vi "multiplier color to multiplier value converter.vi"(2 "mult color":T1) -> (6 "multiplier":dbl)   [LabVIEW 2018]
uses:
  Multiplier--control.ctl
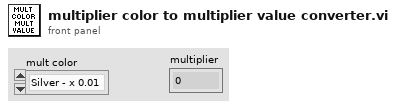
[diagram p1: front panel]
types:
  T1 = typedef "Multiplier--control.ctl" = enum16{"Silver - x 0.01", "Gold - x 0.1 ", "Black - x 1", "Brown - x 10", "Red - x 100", "Orange - x 1k", "Yellow - x 10k", "Green - 100k", "Blue - x 1M", "Violet - x10 M", "Grey - x 100M", "White - x 1G"}
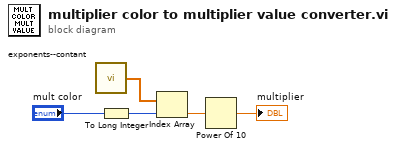
[diagram p0: block diagram]
diagram:
  n1 = call "exponents--contant.vi"() -> ("exponent"=w3:dbl[])  [unwired: 6 in]
  n2 = To Long Integer(number="mult color") -> (32bit integer=w4:i32)
  n3 = Index Array(array=w3, index=w4) -> (element=w2:dbl)
  n4 = Power Of 10(x=w2) -> (10^x=→"multiplier":dbl)
